vi "SSC Digital Configure Time Set Period.vi"(0 "Digital SSC in":T1[](array[typedef]), 5 "time set":string caption="Time Set", 7 "Period (s)":dbl, 11 "error in":errorcluster) -> (4 "Digital SSC out":T1[](array[typedef]), 15 "error out":errorcluster)   [LabVIEW 2019]
doc: "Configures the tset period."
uses:
  SSC Digital.ctl
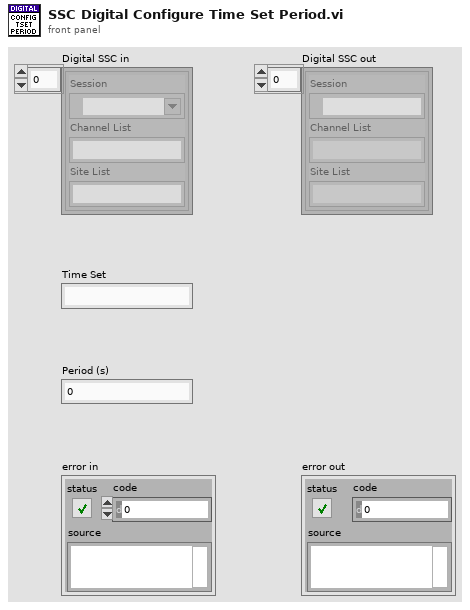
[diagram p1: front panel]
types:
  T1 = typedef "SSC Digital.ctl" = cluster{"Session":refnum<k15>, "Channel List":string, "Site List":string}
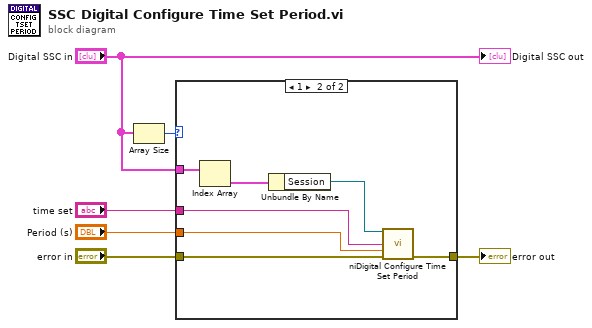
[diagram p0: block diagram]
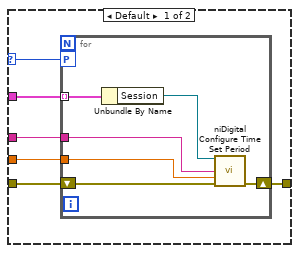
[diagram p2: hidden frame]
diagram:
  n1 = Array Size(array="Digital SSC in") -> (size(s)=w4:i32)
  n2 = case shown="1" w4 {
    selector: w4 -> [w12 _]
    tunnel: "error in" -> [w10 w23]
    tunnel: [w7 w22] -> w5
    tunnel: "Digital SSC in" -> [w11 w25]
    tunnel: "Period (s)" -> [w8 w19]
    tunnel: "time set" -> [w9 w20]
    frame Default {
      n3 = for {
        workers-P: w12 -> [_]
        tunnel: w11 -> [w18] mode=indexing
        tunnel: w9 -> [w14]
        tunnel: w8 -> [w15]
        shift-right: [w16] -> w7
        shift-left: w10 -> [w17]
        n4 = Unbundle By Name(w18) -> ("Session"=w13:refnum<k15>)
        n5 = call <instrlib>:"niDigital Configure Time Set Period.vi"("instrument handle"=w13, "time set"=w14, "period (s)"=w15, "error in"=w17) -> ("error out"=w16:errorcluster)  [unwired: 10 in, 1 out]
      }
    }
    frame 1 {
      n6 = Index Array(array=w25) -> (element=w24:T1)  [unwired: 1 in]
      n7 = Unbundle By Name(w24) -> ("Session"=w21:refnum<k15>)
      n8 = call <instrlib>:"niDigital Configure Time Set Period.vi"("instrument handle"=w21, "time set"=w20, "period (s)"=w19, "error in"=w23) -> ("error out"=w22:errorcluster)  [unwired: 10 in, 1 out]
    }
  }
  "error out" <- w5
  "Digital SSC out" <- "Digital SSC in"
